vi "Test DI.vi"() -> ()   [LabVIEW 2019]
uses:
  <vilib>/FPGAPlugInAG/cRIO-9035/niLvFpga_Open_cRIO-9035.vi
  <vilib>/rvi/interface/common/dynamic/niFpgaDynamicAddResources.vi
  <vilib>/rvi/interface/common/niFpgaWaitOnOcc.vi
  <vilib>/Utility/error.llb/Error Cluster From Error Code.vi
  <vilib>/rvi/errors/niLvFpgaAdjustHostInterfaceError.vi
  <vilib>/FPGAPlugInAG/Dynamic/niLvFpga_Close_Dynamic.vi
  <vilib>/rvi/interface/nirviOpenFPGA/nirviOpenFPGA.xnode
  FPGA Bitfiles/hydrort_FPGATarget_SandBox_w7YRwWudwc4.lvbitx
  FPGA/SandBox.vi
  <vilib>/rvi/interface/nirviMethod/nirviMethod.xnode
  <vilib>/rvi/interface/nirviCloseFPGA/nirviCloseFPGA.xnode
  <vilib>/FPGAPlugInAG/Dynamic/niLvFpga_ConfigureFifo_Dynamic.vi
  <vilib>/rvi/errors/niLvFpgaMergeErrorWithErrorCode.vi
  <vilib>/FPGAPlugInAG/Dynamic/niLvFpga_StartFifo_Dynamic.vi
  <vilib>/FPGAPlugInAG/Dynamic/niLvFpga_ReadFifo_Dynamic.vi
panel:
  out "String":string
  out "error out":errorcluster
  in  "stop":bool
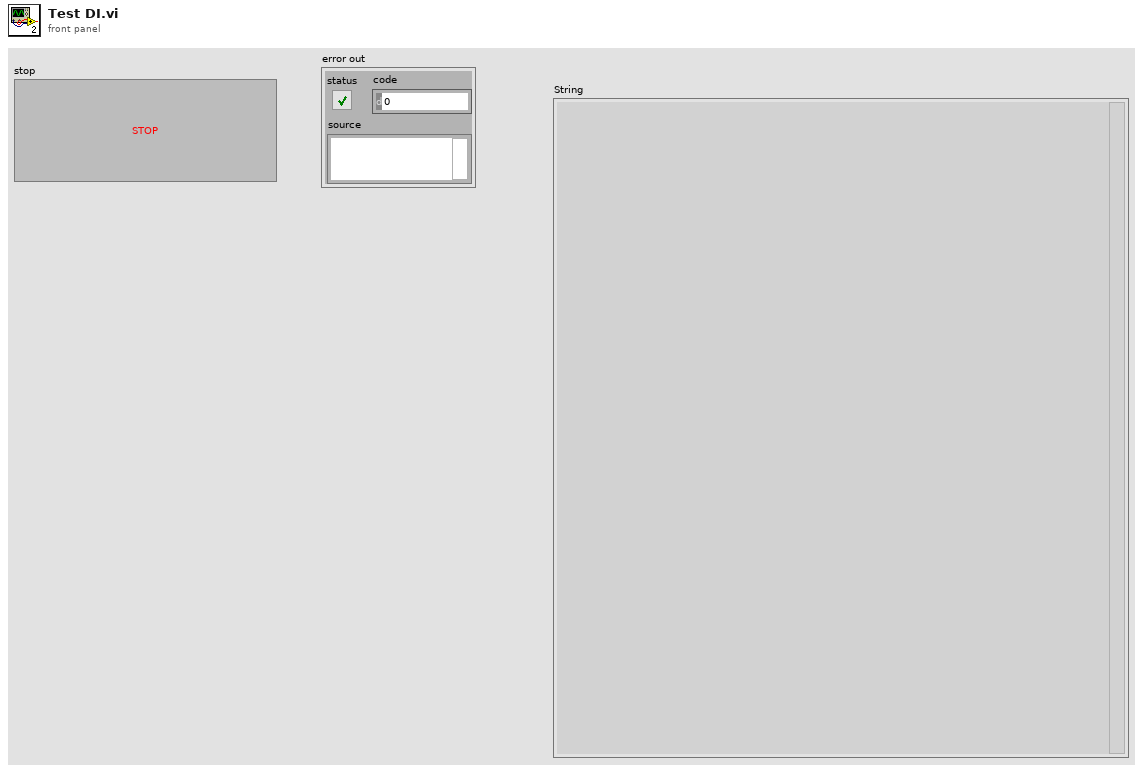
[diagram p1: front panel]
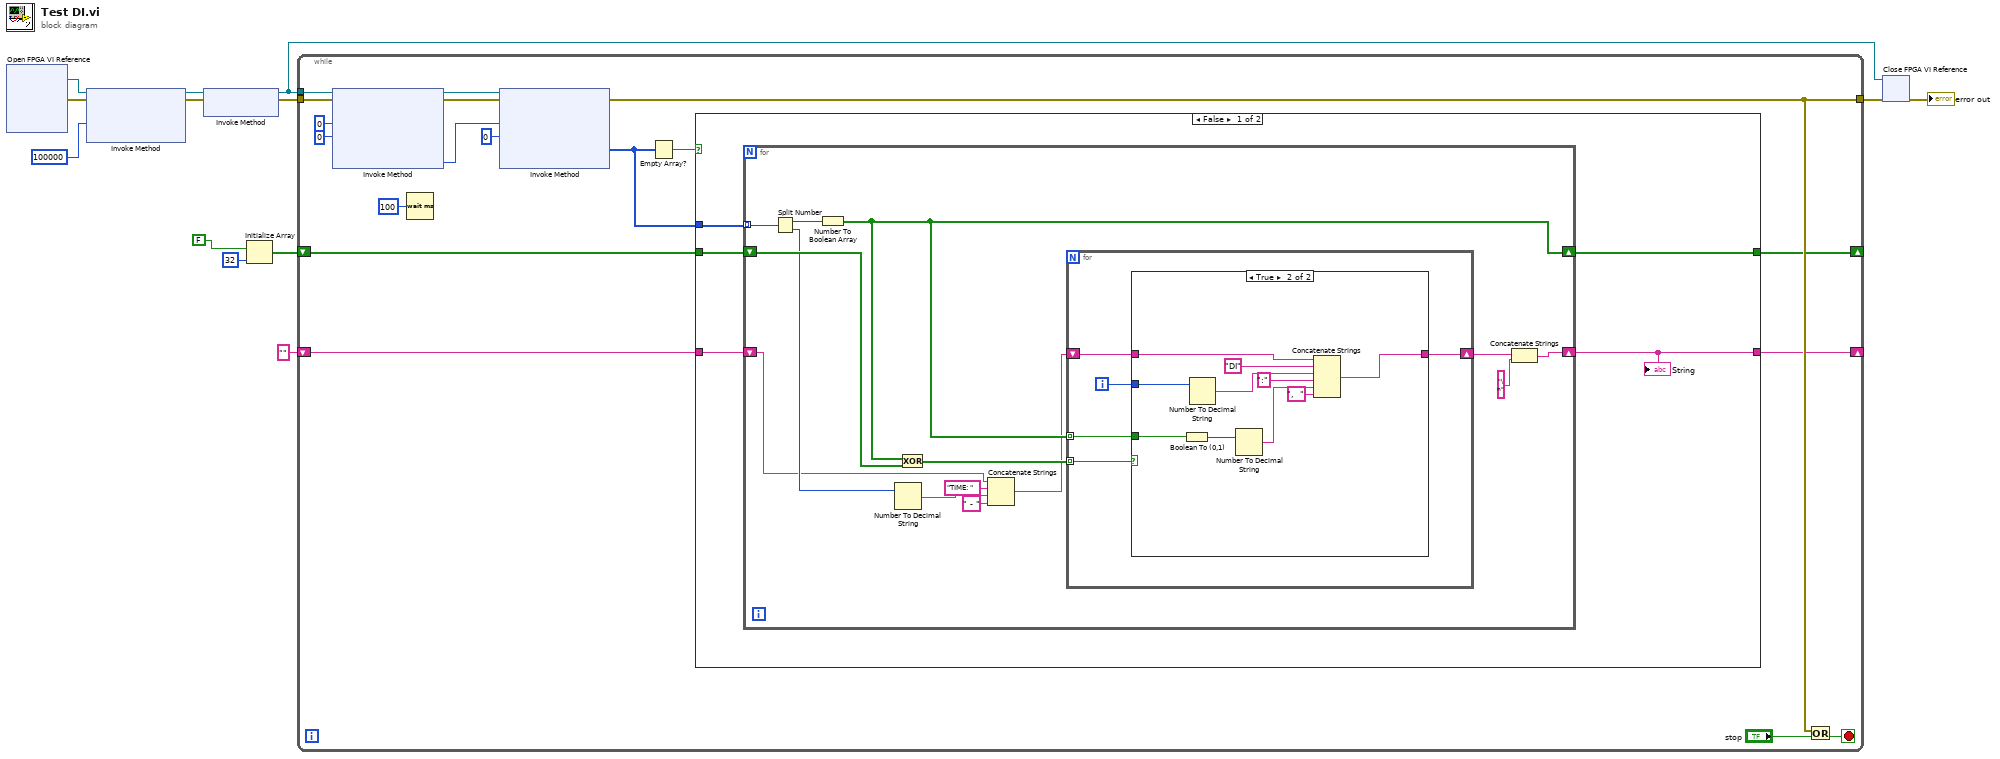
[diagram p0: block diagram]
diagram:
  n1 = xnode "Open FPGA VI Reference"() -> ("FPGA VI Reference Out"=w13:refnum<k20>, "error out"=w11:errorcluster)  [unwired: 2 in]
  n2 = xnode "Invoke Method"("FPGA VI Reference In"=w13, "error in"=w11, "Requested Depth"=u32 100000) -> ("FPGA VI Reference Out"=w10:refnum<k20>, "error out"=w9:errorcluster)  [unwired: 1 out]
  n3 = xnode "Invoke Method"("FPGA VI Reference In"=w10, "error in"=w9) -> ("FPGA VI Reference Out"=w7:refnum<k20>, "error out"=w8:errorcluster)
  n4 = Initialize Array(FALSE, 32 ("dimension size")) -> (w3:bool[])
  n5 = while {
    tunnel: w7 -> [w30]
    tunnel: w8 -> [w29]
    tunnel: [w20] -> w6
    shift-right: [w17] -> _
    shift-left: w3 -> [w16]
    shift-right: [w15] -> _
    shift-left: "" -> [w14]
    stop <- w21 stop-if-true
    n6 = xnode "Invoke Method"("FPGA VI Reference In"=w30, "error in"=w29, "Number of Elements"=u32 0, "Timeout (ms)"=0) -> ("FPGA VI Reference Out"=w26:refnum<k20>, "error out"=w25:errorcluster, "Elements Remaining"=w24:u32)  [unwired: 1 out]
    n7 = Wait (ms)(milliseconds to wait=u32 100) -> ()  [unwired: 1 out]
    n8 = xnode "Invoke Method"("FPGA VI Reference In"=w26, "error in"=w25, "Number of Elements"=w24, "Timeout (ms)"=0) -> ("error out"=w20:errorcluster, "Data"=w18:u64[])  [unwired: 2 out]
    n9 = Empty Array?(array=w18) -> (empty?=w19:bool)
    n10 = case shown="False" w19 {
      tunnel: w18 -> [w36 _]
      tunnel: [w35 w67] -> w17
      tunnel: w16 -> [w34 w67]
      tunnel: [w33 w68] -> w15
      tunnel: w14 -> [w32 w68]
      frame False {
        n11 = for {
          tunnel: w36 -> [w50] mode=indexing
          shift-right: [w46] -> w35
          shift-left: w34 -> [w48]
          shift-right: [w43] -> w33
          shift-left: w32 -> [w38]
          n12 = Split Number(x=w50) -> (hi(x)=w49:u32, lo(x)=w42:u32)
          n13 = Number To Boolean Array(number=w49) -> (Boolean array=w46:bool[])
          n14 = Number To Decimal String(number=w42) -> (decimal integer string=w41:string)  [unwired: 1 in]
          n15 = Exclusive Or(1:w48, 2:w46) -> (0:w47:bool[])
          n16 = Concatenate Strings(w38, "TIME: " ("string"), w41, " - " ("string")) -> (w37:string)
          n17 = for {
            tunnel: w47 -> [w55] mode=indexing
            tunnel: w46 -> [w53] mode=indexing
            shift-right: [w51] -> w45
            shift-left: w37 -> [w52]
            i -> [w54]
            n18 = case shown="True" w55 {
              tunnel: w54 -> [_ w66]
              tunnel: w53 -> [_ w62]
              tunnel: w52 -> [w56 w59]
              tunnel: [w56 w57] -> w51
              frame False {
              }
              frame True {
                n19 = Boolean To (0,1)(Boolean=w62) -> (0, 1=w61:i16)
                n20 = Number To Decimal String(number=w66) -> (decimal integer string=w64:string)  [unwired: 1 in]
                n21 = Number To Decimal String(number=w61) -> (decimal integer string=w60:string)  [unwired: 1 in]
                n22 = Concatenate Strings(w59, "DI" ("string"), w64, ":" ("string"), w60, ",  " ("string")) -> (w57:string)
              }
            }
          }
          n23 = Concatenate Strings(w45, "\n" ("string")) -> (w43:string)
        }
        "String" <- w33
      }
      frame True {
      }
    }
    n24 = Or(x=w20, y="stop") -> (x .or. y?=w21:bool)
  }
  n25 = xnode "Close FPGA VI Reference"("FPGA VI Reference In"=w7, "error in"=w6) -> ("error out"=→"error out":errorcluster)
